vi "SubVI Tester.vi"() -> ()   [LabVIEW 2014]
uses:
  Weather Data.ctl
panel:
  out "气象数据输出":T1={"当前温度"=0.0, "最高温度"=0.0, "最低温度"=0.0, "温度警告？"=FALSE, "温度警告文本"="无警告", "单位"=0} {"单位" items=["摄氏", "华氏"]}
  in  "最低温度":dbl=10.0
  in  "最高温度":dbl=30.0
  in  "停止":bool
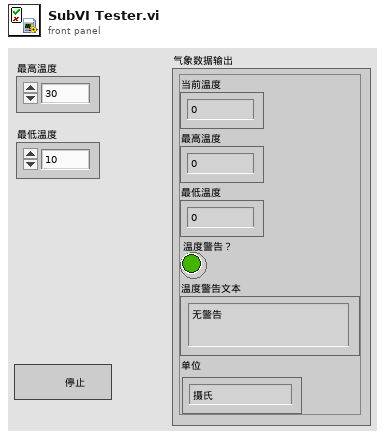
[diagram p1: front panel]
types:
  T1 = typedef "Weather Data.ctl" = cluster{"当前温度":dbl, "最高温度":dbl, "最低温度":dbl, "温度警告？":bool, "温度警告文本":string, "单位":u16}
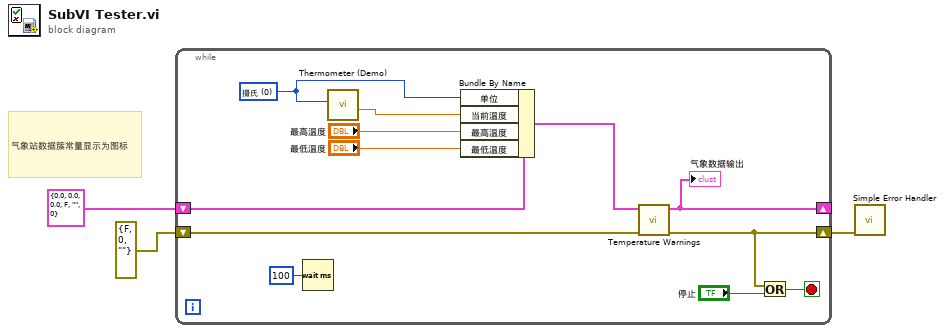
[diagram p0: block diagram]
diagram:
  # "气象站数据簇常量显示为图标"
  n1 = while {
    shift-right: [w6] -> _
    shift-left: T1 {"当前温度"=0.0, "最高温度"=0.0, "最低温度"=0.0, "温度警告？"=FALSE, "温度警告文本"="", "单位"=0} ("气象数据输入") -> [w15]
    shift-right: [w5] -> w2
    shift-left: cluster{"状态":bool, "代码":i32, "源":string} {"状态"=FALSE, "代码"=0, "源"=""} ("错误输出") -> [w11]
    stop <- w12 stop-if-true
    w4 = u16 0 items=["摄氏", "华氏"] ("单位（0：摄氏）")
    n2 = Wait (ms)(milliseconds to wait=u32 100 ("等待时间（毫秒）")) -> ()  [unwired: 1 out]
    n3 = call "Thermometer (Demo).vi"("单位（0：摄氏度）"=w4) -> ("温度值"=w7:dbl)  [unwired: 10 in]
    n4 = Bundle By Name(cluster=w15, "单位"=w4, "当前温度"=w7, "最高温度"="最高温度", "最低温度"="最低温度") -> (w10:T1)
    n5 = call "Temperature Warnings.vi"("错误输入"=w11, "气象数据输入"=w10) -> ("错误输出"=w5:cluster{"状态":bool, "代码":i32, "源":string}, "气象数据输出"=w6:T1)  [unwired: 8 in]
    "气象数据输出" <- w6
    n6 = Or(x=w5, y="停止") -> (x .or. y?=w12:bool)
  }
  n7 = call <vilib>:"Simple Error Handler.vi"("error in (no error)"=w2) -> ()  [unwired: 4 in, 5 out]
